vi "NaN_Index.vi"(10 "Index":i32, 11 "Input":dbl[][](array[numeric])) -> (2 "Index Out":i32, 3 "Output":dbl[](array[numeric]))   [LabVIEW 2019, in "Zen Analytics.lvlib" / "Zen Analytics.lvclass"]
uses:
  Zen Analytics.lvclass
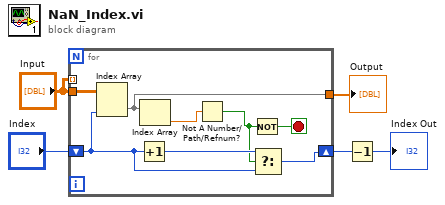
[diagram p0: block diagram]
diagram:
  n1 = for {
    tunnel: "Input" -> [w13]
    tunnel: [w9] -> w1
    shift-right: [w10] -> w3
    shift-left: "Index" -> [w11]
    tunnel: "Input" -> [_] mode=indexing
    stop <- w6 stop-if-true
    n2 = Index Array(array=w13, index (col)=w11) -> (element=w9:dbl[])  [unwired: 1 in]
    n3 = Increment(x=w11) -> (x+1=w12:i32)
    n4 = Index Array(array=w9) -> (element=w8:dbl)  [unwired: 1 in]
    n5 = Not A Number/Path/Refnum?(number/path/refnum=w8) -> (NaN/Path/Refnum?=w7:bool)
    n6 = Not(x=w7) -> (.not. x?=w6:bool)
    n7 = Select(t=w12, s=w7, f=w11) -> (s? t:f=w10:i32)
  }
  "Output" <- w1
  n8 = Decrement(x=w3) -> (x-1=→"Index Out":i32)
